vi "Get Measurement Default Template.vi"(8 "error in":errorcluster, 10 "configuration_defaults":T3, 11 "gRPCid in":T2) -> (0 "error out":errorcluster, 2 "default value":T1, 3 "gRPCid out":u64)   [LabVIEW 2021, in "Default Value Template.lvlib"]
uses:
  Default Value Template.lvlib
  <vilib>/gRPC/Generated APIs/ni/measurementlink/measurement/v2/RPC Messages/google_protobuf_Any.ctl
  <vilib>/gRPC/LabVIEW gRPC Library/Shared/grpcId.ctl
  Configuration.ctl
  92ca8a35-dbcd-4818-a83e-307f6958da28.vi
  <vilib>/gRPC/LabVIEW gRPC Library/Server API/Translate Protobuf Error.vi
  <vilib>/AdvancedString/1D String Array to Delimited String.vi
  <vilib>/gRPC/LabVIEW gRPC Library/Server API/Server/Get Server DLL Path.vi
  <vilib>/gRPC/LabVIEW gRPC Library/grpc-lvsupport-release.lvlib
  <vilib>/gRPC/Generated APIs/ni/measurementlink/measurement/v2/ni.measurementlink.measurement.v2.api.lvlib
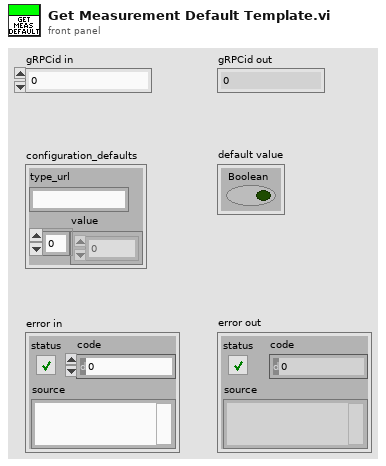
[diagram p1: front panel]
types:
  T1 = typedef "Default Value Template.lvlib/Configuration.ctl" = cluster{"Boolean":bool}
  T2 = typedef "grpc-lvsupport-release.lvlib/grpcId.ctl" = u64
  T3 = typedef "ni.measurementlink.measurement.v2.api.lvlib/google_protobuf_Any.ctl" = cluster{"type_url":string, "value":u8[]}
  T4 = typedef "grpc-lvsupport-release.lvlib/Enum Metadata.ctl" = cluster{"Version":i32, "Name":string, "Type Url":string, "Enum Values":string, "Allow Alias":bool}
  T5 = typedef "grpc-lvsupport-release.lvlib/Message Metadata.ctl" = cluster{"Version":i32, "Name":string, "Type Url":string, "Elements":T6[], "Has Oneof":bool}
  T6 = typedef "grpc-lvsupport-release.lvlib/Message Element Metadata.ctl" = cluster{"Field Name":string, "Embedded Message Name":string, "Protobuf Index":i32, "MessageElementType":T7, "Repeated":bool, "Is in Oneof":bool, "Oneof Container Name":string}
  T7 = typedef "grpc-lvsupport-release.lvlib/Message Element Type.ctl" = enum32{"Int32Value", "FloatValue", "DoubleValue", "BoolValue", "StringValue", "MessageValue", "Int64Value", "UInt32Value", "UInt64Value", "EnumValue", "Bytes", "Fixed64", "Fixed32", "SFixed64", "SFixed32", "SInt64", "SInt32"}
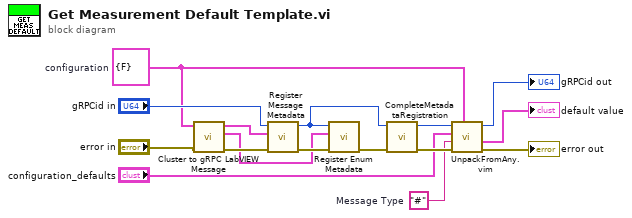
[diagram p0: block diagram]
diagram:
  w6 = T1 {"Boolean"=FALSE}  # configuration
  w8 = "#"  # Message Type
  n1 = call <vilib>:"Cluster to gRPC LabVIEW Message.vi"("error in"="error in", "Cluster"=w6) -> ("error out"=w16:errorcluster, "gRPC Enum Metadata out"=w2:T4[], "gRPC Message Metadata []"=w5:T5[])  [unwired: 7 in]
  n2 = call <vilib>:"Register Message Metadata.vi"("error in"=w16, "Messages"=w5, "gRPCid in"="gRPCid in") -> ("error out"=w4:errorcluster, "gRPCid out"=w1:T2)  [unwired: 7 in]
  n3 = call <vilib>:"Register Enum Metadata.vi"("error in"=w4, "Enum Metadata"=w2, "gRPCid in"=w1) -> ("error out"=w3:errorcluster)  [unwired: 7 in, 1 out]
  n4 = call <vilib>:"CompleteMetadataRegistration.vi"("error in"=w3, "gRPC ID in"=w1) -> ("error out"=w14:errorcluster, "gRPC ID Out"=w15:T2)  [unwired: 8 in]
  n5 = call "UnpackFromAny.vim"("Data Type"=w6, "error in"=w14, "Message Type"=w8, "Any"="configuration_defaults", "gRPCid in"=w15) -> ("error out"=→"error out":errorcluster, "Unpacked Value"=→"default value":T1, "gRPCid out"=→"gRPCid out":u64)  [unwired: 4 in]
